vi "testDestroy.vi"(8 "error in (no error)":errorcluster, 11 "TestCase in":refnum<class "ObjectList_Delegations.lvclass">) -> (0 "error out":errorcluster, 3 "TestCase out":refnum<class "ObjectList_Delegations.lvclass">)   [LabVIEW 2013, in "ObjectList_Delegations.lvclass"]
uses:
  ObjectList_Delegations.lvclass
  ObjectList_Delegations.lvclass/ObjectList_Delegations.ctl
  source/LapDog.Collections.Lists/ObjectList/ObjectList.lvclass
  <vilib>/addons/_JKI Toolkits/VI Tester/TestCase.llb/TestCase.lvclass
  UnitTestComparisons/UnitTestComparisons.lvlib
  Test Doubles/ListImp_RefSpy/ListImp_RefSpy.lvclass
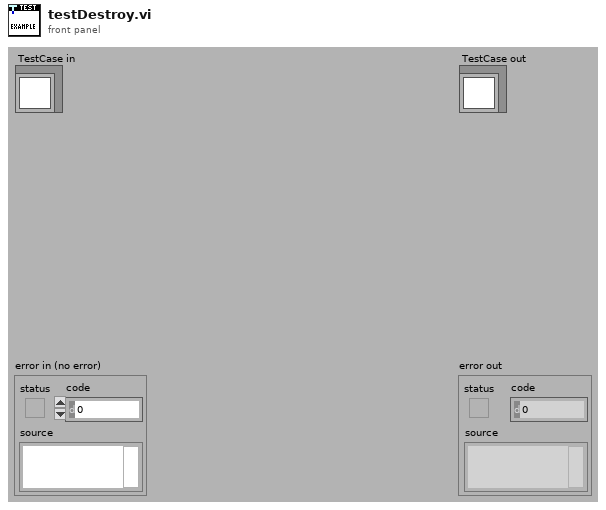
[diagram p1: front panel]
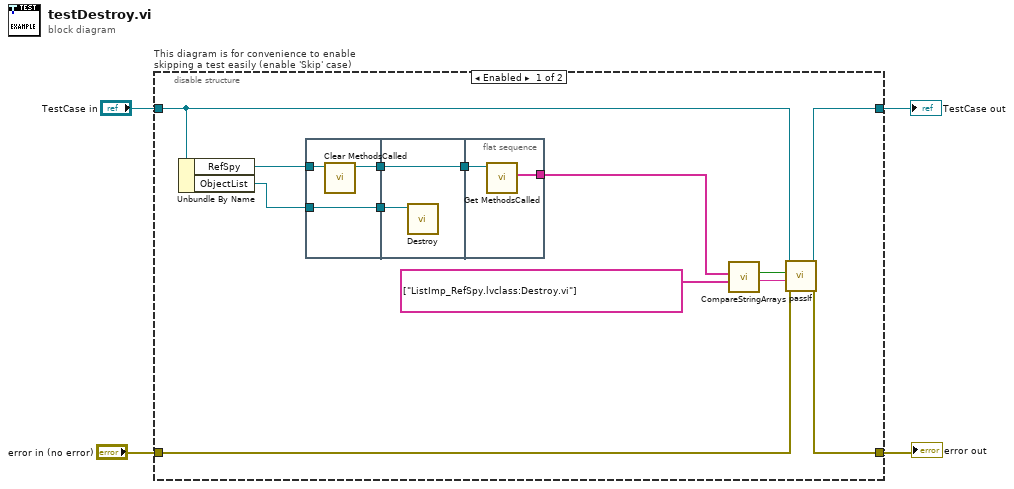
[diagram p0: block diagram]
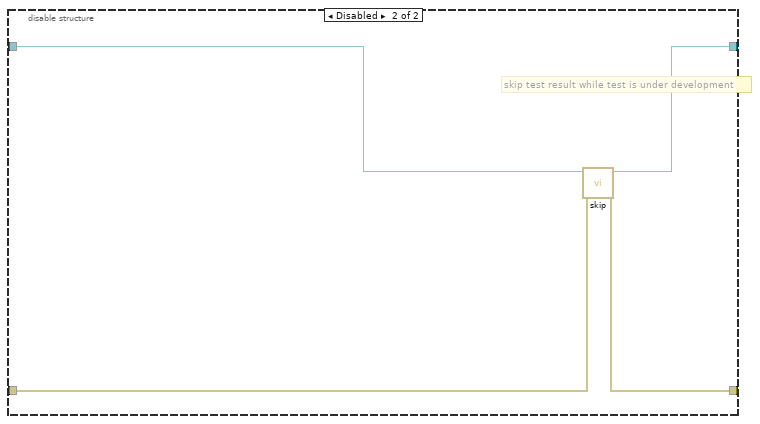
[diagram p2: hidden frame]
diagram:
  n1 = disable-structure "This diagram is for convenience to enable skipping a test easily (enable 'Skip' case)" shown="Enabled" {
    disable-tunnel: "TestCase in" -> [w12 w28]
    disable-tunnel: [w17 w26] -> w1
    disable-tunnel: [w16 w27] -> w3
    disable-tunnel: "error in (no error)" -> [w15 w25]
    frame Enabled {
      n2 = Unbundle By Name(w12) -> ("RefSpy"=w9:refnum<class "ListImp_RefSpy.lvclass">, "ObjectList"=w11:refnum<class "ObjectList.lvclass">)
      n3 = flat-sequence {
        tunnel: w9 -> [w19]
        tunnel: w11 -> [w20]
        tunnel: [w20] -> w6
        tunnel: [w18] -> w5
        tunnel: [w22] -> w10
        tunnel: w6 -> [w21]
        tunnel: w5 -> [w22]
        tunnel: w10 -> [w24]
        tunnel: [w23] -> w7
        frame #0 {
          n4 = call "Clear MethodsCalled.vi"("MockListImp in"=w19) -> ("MockListImp out"=w18:refnum<class "ListImp_RefSpy.lvclass">)  [unwired: 9 in, 1 out]
        }
        frame #1 {
          n5 = call-dynamic "Destroy.vi"("List in"=w21) -> ()  [unwired: 10 in, 1 out]
        }
        frame #2 {
          n6 = call "Get MethodsCalled.vi"("MockListImp"=w24) -> ("MethodsCalled"=w23:string[])  [unwired: 9 in, 1 out]
        }
      }
      n7 = call "CompareStringArrays.vi"("Expected Strings"=string[] ["ListImp_RefSpy.lvclass:Destroy.vi"] ("Actual Strings"), "Actual Strings"=w7) -> ("Message"=w13:string, "Equal?"=w14:bool)  [unwired: 8 in]
      n8 = call-dynamic "passIf.vi"("error in (no error)"=w15, "message (\"\")"=w13, "pass"=w14, "TestCase in"=w12) -> ("error out"=w16:errorcluster, "TestCase out"=w17:refnum<class "ObjectList_Delegations.lvclass">)  [unwired: 6 in]
    }
    frame Disabled {
      # "skip test result while test is under development"
      n9 = call <vilib>:"skip.vi"("error in (no error)"=w25, "TestCase in"=w28) -> ("error out"=w27:errorcluster, "TestCase out"=w26:refnum<class "ObjectList_Delegations.lvclass">)  [unwired: 8 in]
    }
  }
  "error out" <- w3
  "TestCase out" <- w1
